vi "oax_gsUpdate Status String.vi"(4 "error in (no error)":errorcluster, 5 "old status":string, 6 "new status":string, 7 "Ctl Refnum":refnum<vi>) -> (0 "error out":errorcluster)   [LabVIEW 2017]
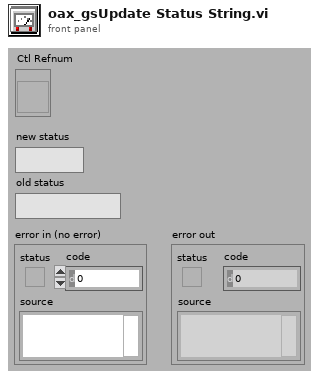
[diagram p1: front panel]
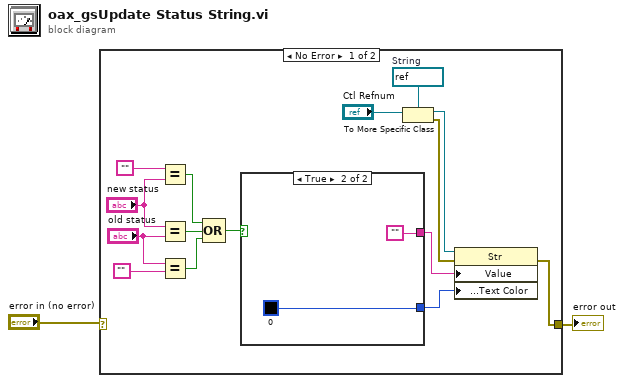
[diagram p0: block diagram]
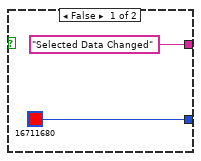
[diagram p2: hidden frame]
diagram:
  n1 = case shown="No Error" "error in (no error)" {
    selector: "error in (no error)" -> [_ w22]
    tunnel: [w11 w22] -> w1
    frame No Error {
      w14 = refnum<vi> refnum  # String
      n2 = Equal?(x="", y="new status") -> (x = y?=w3:bool)
      n3 = Equal?(x="new status", y="old status") -> (x = y?=w6:bool)
      n4 = Equal?(x="old status", y="") -> (x = y?=w4:bool)
      n5 = Compound Arithmetic op=OR(w3, w6, w4) -> (w5:bool)
      n6 = case shown="True" w5 {
        tunnel: ["Selected Data Changed" ""] -> w17
        tunnel: [u32 16711680 u32 0] -> w13
        frame False {
        }
        frame True {
        }
      }
      n7 = To More Specific Class(target class=w14, reference="Ctl Refnum") -> (specific class reference=w15:refnum<vi>, error out=w12:errorcluster)  [unwired: 1 in]
      n8 = property class="Str"(reference=w15, error in=w12, "Value"=w17, "Text.Text Colors:Text Color"=w13) -> (error out=w11:errorcluster)  [unwired: 1 out]
    }
    frame Error {
    }
  }
  "error out" <- w1
